vi "Read Hydrogen PPM.vi"(0 "Session Handle in":T1, 11 "error in (no error)":errorcluster) -> (4 "Session Handle out":T1, 6 "H2 PPM":dbl, 8 "Seconds Updated":dbl, 15 "error out":errorcluster)   [LabVIEW 2015, in "Gas.lvclass"]
uses:
  Gas.lvclass
  Typedefs/Session Handle.ctl
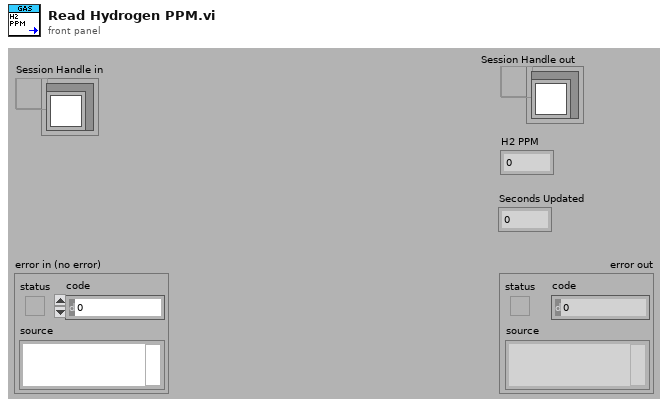
[diagram p1: front panel]
types:
  T1 = typedef "Gas.lvclass/Session Handle.ctl" = refnum<data-value>
  T2 = typedef "XNET Frame CAN.ctl" = cluster{"timestamp":timestamp, "payload":u8[], "identifier":u32, "type":T3, "extended?":bool, "echo?":bool}
  T3 = typedef "XNET Frame Type CAN.ctl" = u8
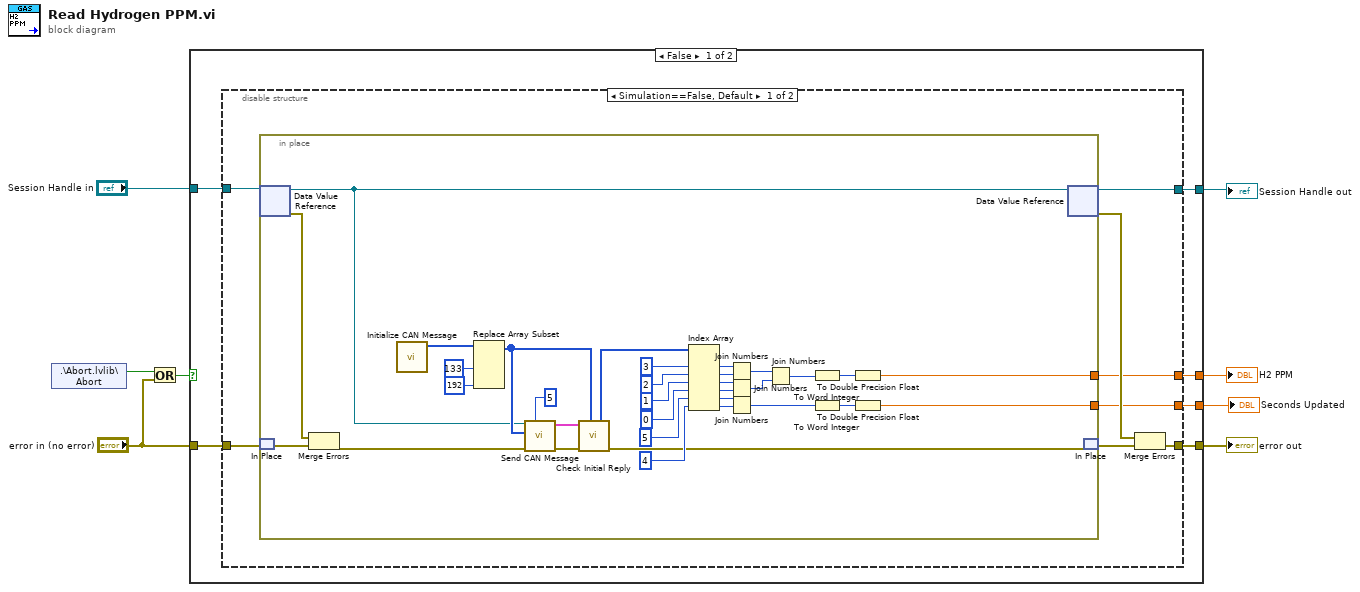
[diagram p0: block diagram]
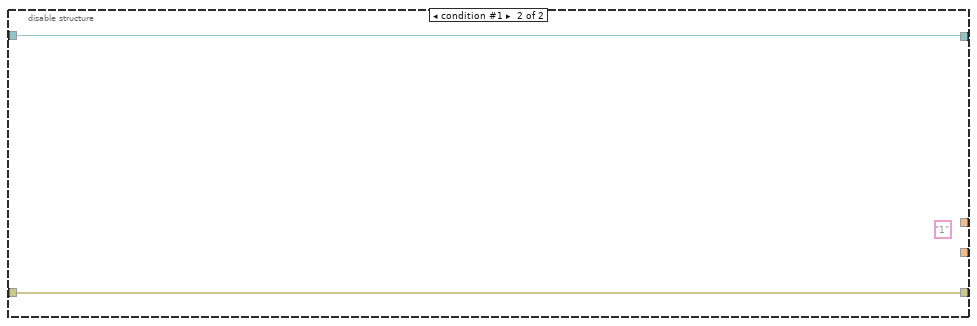
[diagram p2: hidden frame]
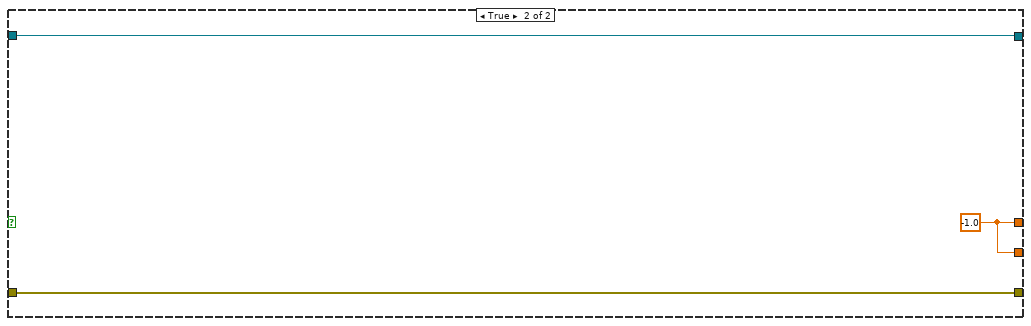
[diagram p3: hidden frame]
diagram:
  n1 = shared-variable ".\\Abort.lvlib\\Abort"() -> (w5:bool)  [unwired: 1 in, 1 out]
  n2 = Or(x=w5, y="error in (no error)") -> (x .or. y?=w3:bool)
  n3 = case shown="False" w3 {
    tunnel: [w14 w60] -> w7
    tunnel: [w13 w59] -> w6
    tunnel: "Session Handle in" -> [w12 w60]
    tunnel: "error in (no error)" -> [w11 w59]
    tunnel: [w10 w58] -> w2
    tunnel: [w9 w58] -> w1
    frame False {
      n4 = disable-structure shown="Simulation==False, Default" {
        disable-tunnel: [w22 w57] -> w14
        disable-tunnel: [w19 w56] -> w13
        disable-tunnel: w12 -> [w18 w57]
        disable-tunnel: w11 -> [w17 w56]
        disable-tunnel: [w16 _] -> w10
        disable-tunnel: [w15 _] -> w9
        frame condition #0 (active) {
          n5 = in-place {
            in-place-border: [w45] -> w16
            in-place-border: [w25] -> w15
            n6 = in-place-dvr #1(w18) -> (w44:refnum<class "Gas.lvclass">, w51:errorcluster)
            n7 = in-place-match #2(w17) -> (w50:errorcluster)
            n8 = Merge Errors(w51, w50) -> (w43:errorcluster)
            n9 = call "Initialize CAN Message.vi"() -> ("Initial Payload"=w53:u8[])  [unwired: 11 in]
            n10 = Replace Array Subset(array=w53, new element #1=u8 133 ("new element/subarray"), new element #2=u8 192 ("new element/subarray")) -> (w49:u8[])  [unwired: 2 in]
            n11 = call "Send CAN Message.vi"("Number of Retries"=5, "error in (no error)"=w43, "payload"=w49, "Gas In"=w44) -> ("error out"=w24:errorcluster, "Reply"=w47:T2[])  [unwired: 5 in, 1 out]
            n12 = call "Check Initial Reply.vi"("Write Message"=w49, "error in (no error)"=w24, "Reply"=w47) -> ("error out"=w23:errorcluster, "Data Packet"=w52:u8[])  [unwired: 5 in, 2 out]
            n13 = Index Array(array=w52, index #1=3 ("index"), index #2=2 ("index"), index #3=1 ("index"), index #4=0 ("index"), index #5=5 ("index"), index #6=4 ("index")) -> (element #1=w36:u8, element #2=w35:u8, element #3=w34:u8, element #4=w33:u8, element #5=w32:u8, element #6=w31:u8)
            n14 = Join Numbers(hi=w36, lo=w35) -> ((hi.lo)=w30:u16)
            n15 = Join Numbers(hi=w34, lo=w33) -> ((hi.lo)=w29:u16)
            n16 = Join Numbers(hi=w32, lo=w31) -> ((hi.lo)=w26:u16)
            n17 = Join Numbers(hi=w30, lo=w29) -> ((hi.lo)=w28:u32)
            n18 = To Word Integer(number=w28) -> (16bit integer=w46:i16)
            n19 = To Word Integer(number=w26) -> (16bit integer=w27:i16)
            n20 = To Double Precision Float(number=w46) -> (double precision float=w45:dbl)
            n21 = To Double Precision Float(number=w27) -> (double precision float=w25:dbl)
            n22 = in-place-dvr #1(w44) -> (w22:T1, w20:errorcluster)
            n23 = in-place-match #2(w23) -> (w21:errorcluster)
          }
          n24 = Merge Errors(w20, w21) -> (w19:errorcluster)
        }
        frame condition #1 {
          (unwired) "1"
        }
      }
    }
    frame True {
      w58 = -1.0
    }
  }
  "Session Handle out" <- w7
  "error out" <- w6
  "H2 PPM" <- w2
  "Seconds Updated" <- w1
